vi "Test Broadcast State Data.vi"(8 "error in (no error)":errorcluster, 11 "Test Case In":refnum<class "Debugger Test.lvclass">) -> (0 "error out":errorcluster, 3 "Test Case Out":refnum<class "Debugger Test.lvclass">)   [LabVIEW 2020]
uses:
  Debugger Test.lvclass/Debugger Test.ctl
  01074fa8-ee8a-411d-bc8b-fc92c4f90959.vi
  source/Process/Debug Process.lvclass
  source/Debugger/Debugger.lvclass
  C:/Users/anton/Documents/GitHub/triarc-debugger/source/Process/Debug Process.lvclass
  C:/Users/anton/Documents/GitHub/triarc-debugger/source/Debugger/Debugger.lvclass
  C:/Users/anton/Documents/GitHub/triarc-debugger/source/Debug Data Event/Debug Data Listener.lvclass
  source/Debug Data/Debug Data.lvclass
  source/Debug Data/Raw Debug Data.ctl
  <vilib>/Astemes/Triarc Framework/Broadcast Event Helpers/Broadcast Event Helpers.lvlib
  Debugger Test.lvclass
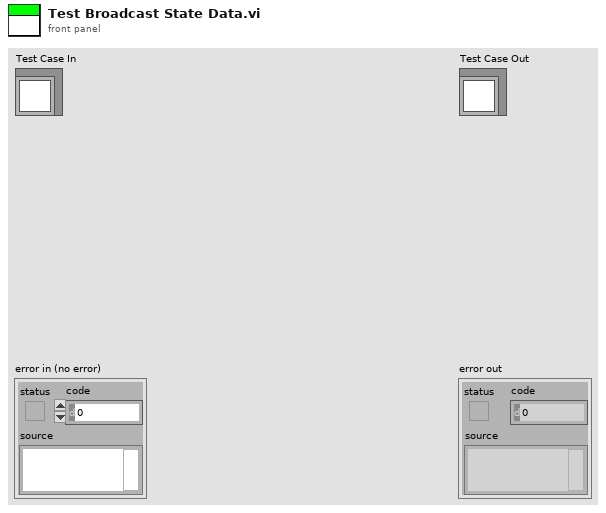
[diagram p1: front panel]
types:
  T1 = typedef "Debug Data.lvclass/Raw Debug Data.ctl" = cluster{"Action":string, "Call Chain":string, "Process":string, "Message":string, "Message Data":variant, "Time":dbl}
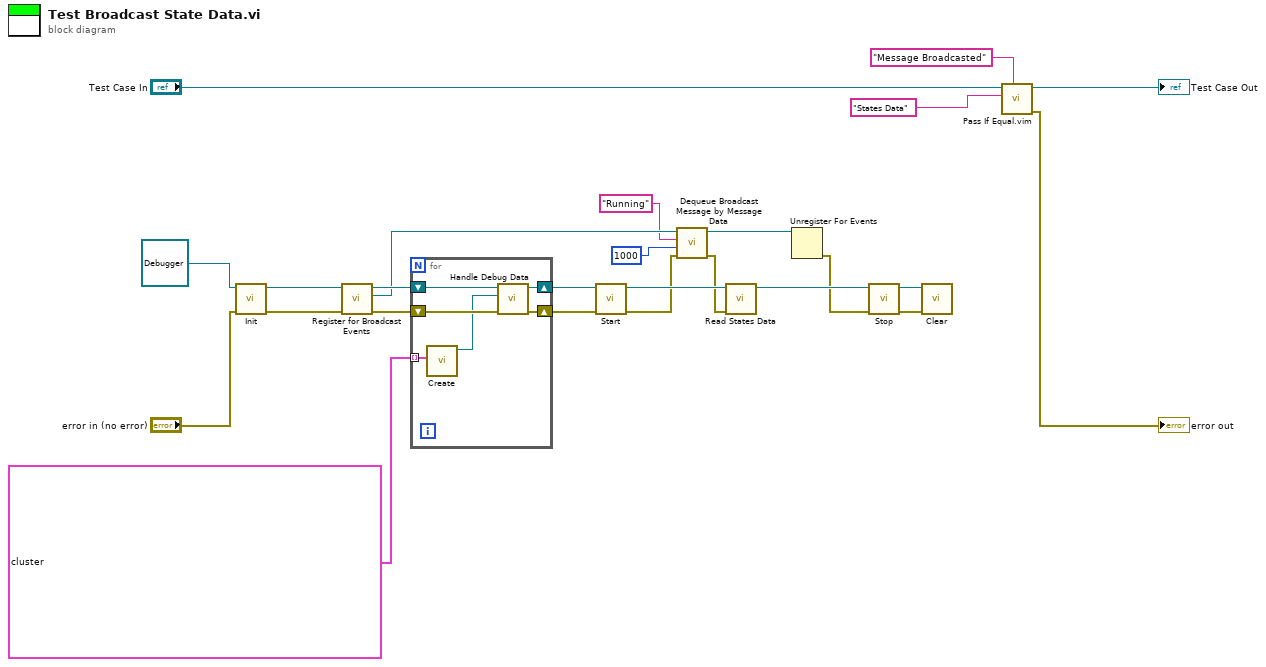
[diagram p0: block diagram]
diagram:
  n1 = call-dynamic "Init.vi"("error in (no error)"="error in (no error)", "Process In"=refnum<class "Debugger.lvclass"> refnum ("Debug Data Event In 2")) -> ("error out"=w12:errorcluster, "Process Out"=w13:refnum<class "Debugger.lvclass">)  [unwired: 8 in]
  n2 = call "Register for Broadcast Events.vi"("error in (no error)"=w12, "Process In"=w13) -> ("error out"=w23:errorcluster, "Event Registration Refnum Out"=w9:refnum<event-registration>, "Process Out"=w19:refnum<class "Debugger.lvclass">)  [unwired: 7 in]
  n3 = for {
    shift-right: [w29] -> w14
    shift-left: w23 -> [w31]
    shift-right: [w30] -> w11
    shift-left: w19 -> [w28]
    tunnel: T1[] [{"Action"="Send", "Call Chain"="Test.vi:123456", "Process"="Process 1", "Message"="Init", "Message Data"=variant, "Time"=0.0}, {"Action"="Receive", "Call Chain"="TF.lvlib:Process.lvclass:Handle Messages.vi:1960001", "Process"="Process 1", "Message"="Init", "Message Data"=variant, "Time"=0.0}, {"Action"="Send", "Call Chain"="Test.vi", "Process"="Process 1", "Message"="Start", "Message Data"=variant, "Time"=0.0}, {"Action"="Receive", "Call Chain"="Test.vi", "Process"="Process 1", "Message"="Start", "Message Data"=variant, "Time"=0.0}] ("Debug Data Cluster") -> [w26] mode=indexing
    n4 = call "Create.vi"("Debug Data Cluster"=w26) -> ("Debug Data out"=w27:refnum<class "Debug Data.lvclass">)  [unwired: 9 in, 1 out]
    n5 = call-dynamic "Handle Debug Data.vi"("error in (no error)"=w31, "Debug Data.lvclass"=w27, "Debug Data Event In"=w28) -> ("error out"=w29:errorcluster, "Debug Data Event Out"=w30:refnum<class "Debugger.lvclass">)  [unwired: 7 in]
  }
  n6 = call "Start.vi"("error in (no error)"=w14, "Process In"=w11) -> ("error out"=w7:errorcluster, "Process Out"=w10:refnum<class "Debugger.lvclass">)  [unwired: 7 in, 1 out]
  n7 = call <vilib>:"Dequeue Broadcast Message by Message Data.vi"("error in (no error)"=w7, "Timeout (-1)"=1000, "Message Data"="Running", "Event Registration Refnum"=w9) -> ("error out"=w6:errorcluster, "Event Registration Refnum Out"=w8:refnum<event-registration>)  [unwired: 3 in, 3 out]
  n8 = call "Read States Data.vi"("error in (no error)"=w6, "Debugger in"=w10) -> ("Debugger in 2"=w22:refnum<class "Debugger.lvclass">)  [unwired: 7 in, 2 out]
  n9 = Unregister For Events(event registration refnum=w8) -> (error out=w16:errorcluster)  [unwired: 1 in]
  n10 = call "Stop.vi"("error in (no error)"=w16, "Process In"=w22) -> ("error out"=w20:errorcluster, "Process Out"=w21:refnum<class "Debugger.lvclass">)  [unwired: 7 in, 1 out]
  n11 = call-dynamic "Clear.vi"("error in (no error)"=w20, "Process In"=w21) -> ()  [unwired: 9 in, 1 out]
  n12 = call "Pass If Equal.vim"("Description"="Message Broadcasted", "Expected"="States Data", "LUnit Test Case In"="Test Case In") -> ("error out"=→"error out":errorcluster, "LUnit Test Case Out"=→"Test Case Out":refnum<class "Debugger Test.lvclass">)  [unwired: 7 in]
